vi "Update Status Command.vi"(8 "error in":errorcluster, 10 "Status":T1 {"Monitor Doubles"."4" format="%#_9g"; "Monitor Doubles"."3" format="%#_9g"; "Monitor Doubles"."2" format="%#_9g"; "Monitor Doubles"."1" format="%#_9g"}, 11 "CoreOOB_Tx in":refnum<class "CIFCoreOOB_Tx.lvclass">) -> (0 "error out":errorcluster, 3 "CoreOOB_Tx out":refnum<class "CIFCoreOOB_Tx.lvclass">)   [LabVIEW 2021, in "CIFCoreOOB_Tx.lvclass"]
uses:
  CIFCoreOOB_Tx.lvclass
  D:/dev/CIF-LVCore/src/CIFUtilities/CIFOutOfBand/CIFOutOfBand.lvclass
  CIFCoreCommon/Typedef/Plugin Status.ctl
  CIFCoreCommon/Typedef/Plugin State.ctl
  CIFCoreCommon/Typedef/Timing Statistics.ctl
  CIFCoreCommon/Typedef/Timing Stats Base.ctl
  CIFCoreCommon/Typedef/FIFO Statistics.ctl
  CIFCoreCommon/Typedef/Simple Error.ctl
  CIFCoreCommon/Typedef/Monitor Doubles.ctl
  CIFCoreCommon/Typedef/Monitor U64.ctl
  CIFCoreCommon/Typedef/Monitor I64.ctl
  CIFUtilities/CIFOutOfBand/CIFOutOfBand.lvclass/CIFOutOfBand.ctl
  Typedef/Template Payload.ctl
  CIFCoreCommon/Typedef/Plugin Overrides.ctl
  CIFCoreCommon/Typedef/Timing Overrides.ctl
  Typedef/OOB Core Commands.ctl
  CIFCoreOOB_Tx.lvclass/CIFCoreOOB_Tx.ctl
  CIFUtilities/CIFOutOfBand/CIFOutOfBand.lvclass
  CIFCoreCommon/CIFCoreCommon.lvlib
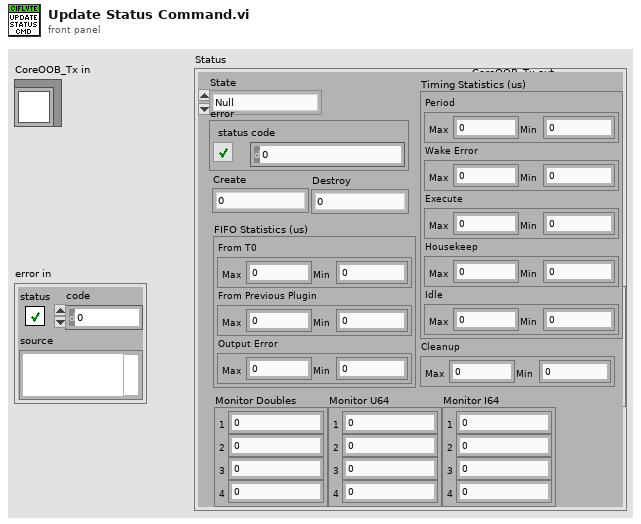
[diagram p1: front panel]
types:
  T1 = typedef "CIFCoreCommon.lvlib/Plugin Status.ctl" = cluster{"State":T2, "Timing Statistics (us)":T3, "FIFO Statistics (us)":T5, "error":T6, "Monitor Doubles":T7, "Monitor U64":T8, "Monitor I64":T9, "Cleanup":T4, "Create":dbl, "Destroy":dbl}
  T2 = typedef "CIFCoreCommon.lvlib/Plugin State.ctl" = enum32{"Null", "Creating", "Listening", "Running", "CleaningUp", "Destroying"}
  T3 = typedef "CIFCoreCommon.lvlib/Timing Statistics.ctl" = cluster{"Period":T4, "Wake Error":T4, "Execute":T4, "Housekeep":T4, "Idle":T4}
  T4 = typedef "CIFCoreCommon.lvlib/Timing Stats Base.ctl" = cluster{"Max":i32, "Min":i32}
  T5 = typedef "CIFCoreCommon.lvlib/FIFO Statistics.ctl" = cluster{"From T0":T4, "From Previous Plugin":T4, "Output Error":T4}
  T6 = typedef "CIFCoreCommon.lvlib/Simple Error.ctl" = cluster{"status":bool, "code":i32}
  T7 = typedef "CIFCoreCommon.lvlib/Monitor Doubles.ctl" = cluster{"1":dbl, "2":dbl, "3":dbl, "4":dbl}
  T8 = typedef "CIFCoreCommon.lvlib/Monitor U64.ctl" = cluster{"1":u64, "2":u64, "3":u64, "4":u64}
  T9 = typedef "CIFCoreCommon.lvlib/Monitor I64.ctl" = cluster{"1":i64, "2":i64, "3":i64, "4":i64}
  T10 = typedef "CIFCoreOOB_Tx.lvclass/Template Payload.ctl" = cluster{"Status":T1, "Plugin Overrides":T11}
  T11 = typedef "CIFCoreCommon.lvlib/Plugin Overrides.ctl" = cluster{"Timing Overrides":T12}
  T12 = typedef "CIFCoreCommon.lvlib/Timing Overrides.ctl" = cluster{"Override Timing":bool, "Period (s)":dbl}
  T13 = typedef "CIFCoreOOB_Tx.lvclass/OOB Core Commands.ctl" = enum8{"Status", "Overrides"}
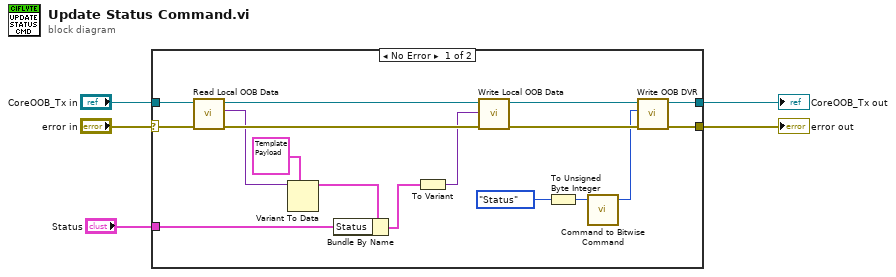
[diagram p0: block diagram]
diagram:
  n1 = case shown="No Error" "error in" {
    selector: "error in" -> [w20 w24]
    tunnel: [w21 w24] -> w4
    tunnel: "CoreOOB_Tx in" -> [w19 w23]
    tunnel: [w22 w23] -> w2
    tunnel: "Status" -> [w6 _]
    frame No Error {
      n2 = call "Read Local OOB Data.vi"("error in"=w20, "OOB in"=w19) -> ("error out"=w10:errorcluster, "Local OOB Data"=w8:variant, "OOB out"=w11:refnum<class "CIFCoreOOB_Tx.lvclass">)  [unwired: 7 in]
      n3 = Variant To Data(type=T10 {"Status"={"State"=enum."Null", "Timing Statistics (us)"={"Period"={"Max"=0, "Min"=1000}, "Wake Error"={"Max"=3, "Min"=2}, "Execute"={"Max"=994, "Min"=992}, "Housekeep"={"Max"=2, "Min"=2}, "Idle"={"Max"=0, "Min"=0}}, "FIFO Statistics (us)"={"From T0"={"Max"=0, "Min"=0}, "From Previous Plugin"={"Max"=0, "Min"=0}, "Output Error"={"Max"=0, "Min"=0}}, "error"={"status"=FALSE, "code"=0}, "Monitor Doubles"={"1"=0.0, "2"=0.0, "3"=0.0, "4"=0.0}, "Monitor U64"={"1"=0, "2"=0, "3"=0, "4"=0}, "Monitor I64"={"1"=0, "2"=0, "3"=0, "4"=0}, "Cleanup"={"Max"=0, "Min"=0}, "Create"=0.0, "Destroy"=0.0}, "Plugin Overrides"={"Timing Overrides"={"Override Timing"=FALSE, "Period (s)"=0.0}}} ("Template Payload"), Variant=w8) -> (data=w13:T10)  [unwired: 1 in, 1 out]
      n4 = Bundle By Name(cluster=w13, "Status"=w6) -> (w12:T10)
      n5 = To Variant(anything=w12) -> (Variant=w9:variant)
      n6 = call "Write Local OOB Data.vi"("error in"=w10, "Local OOB Data"=w9, "OOB in"=w11) -> ("error out"=w18:errorcluster, "OOB out"=w17:refnum<class "CIFCoreOOB_Tx.lvclass">)  [unwired: 7 in]
      n7 = To Unsigned Byte Integer(number=OOB_Core_Commands."Status" ("OOB Main Commands")) -> (unsigned 8bit integer=w16:u8)
      n8 = call "Command to Bitwise Command.vi"("OOB Command"=w16) -> ("bit command"=w15:u64)  [unwired: 3 in]
      n9 = call "Write OOB DVR.vi"("error in"=w18, "Commands (bitwise)"=w15, "OOB in"=w17) -> ("error out"=w21:errorcluster, "OOB out"=w22:refnum<class "CIFCoreOOB_Tx.lvclass">)  [unwired: 7 in]
    }
    frame Error {
    }
  }
  "error out" <- w4
  "CoreOOB_Tx out" <- w2
